vi "Test_MergeErrorsPublication_ErrorCluster_ErrorMerged.vi"(8 "error in (no error)":errorcluster, 11 "TestCase in":refnum<class "TestPublicationPolicy.lvclass">) -> (0 "error out":errorcluster, 3 "TestCase out":refnum<class "TestPublicationPolicy.lvclass">)   [LabVIEW 2017, in "TestPublicationPolicy.lvclass"]
uses:
  TestPublicationPolicy.lvclass
  MergeErrorsPublication/MergeErrorsPublication.lvclass
  C:/Git/mva-framework/Framework/IMediator/IPublicationPolicy/IPublicationPolicy.lvclass
  IMediator/IPublicationPolicy/IPublicationPolicy.lvclass
  Transport/QueueTransport/QueueTransport.lvclass/QueueTransport.ctl
  IMediator/PublishRequest/PublishRequest.lvclass/PublishRequest.ctl
  IMediator/MutexedPublishRequest/MutexedPublishRequest.lvclass/MutexedPublishRequest.ctl
  IMediator/PublishRequest/Write Publish Request Data.vi
  Transport/QueueTransport/QueueTransport.lvclass
  C:/Git/mva-framework/Framework/IMediator/ITransport/ITransport.lvclass
  IMediator/MutexedPublishRequest/MutexedPublishRequest.lvclass
  C:/Git/mva-framework/Framework/IMediator/PublishRequest/PublishRequest.lvclass
  <vilib>/Utility/error.llb/Error Cluster From Error Code.vi
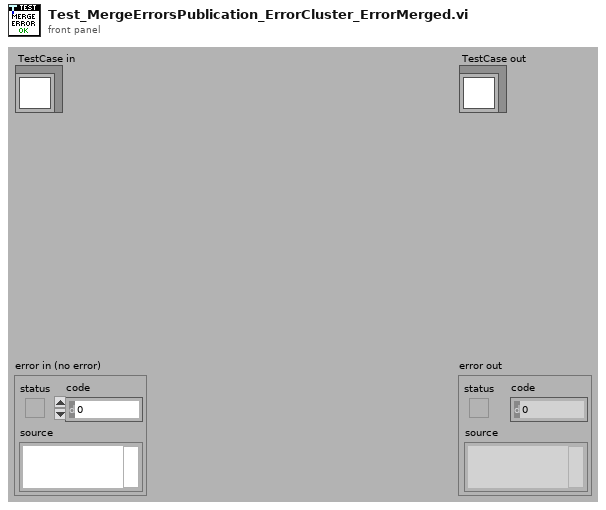
[diagram p1: front panel]
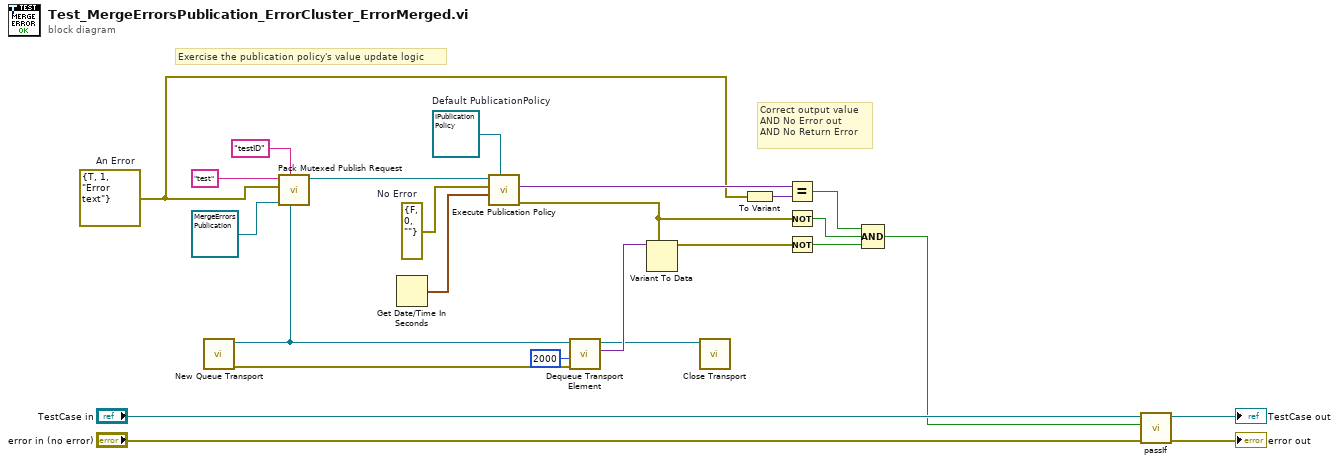
[diagram p0: block diagram]
diagram:
  w2 = errorcluster {"status"=TRUE, "code"=1, "source"="Error text"}  # An Error
  w17 = refnum<class "IPublicationPolicy.lvclass"> refnum  # Default PublicationPolicy
  w21 = errorcluster {"status"=FALSE, "code"=0, "source"=""}  # No Error
  # "Correct output value\nAND No Error out\nAND No Return Error"
  # "Exercise the publication policy's value update logic"
  n1 = call "New Queue Transport.vi"() -> ("error out"=w13:errorcluster, "QueueTransport"=w14:refnum<class "QueueTransport.lvclass">)  [unwired: 10 in]
  n2 = call "Pack Mutexed Publish Request.vi"("Return Error Transport"=w14, "Publisher ID"="testID", "PublicationPolicy"=refnum<class "MergeErrorsPublication.lvclass"> refnum ("PublicationPolicy.lvlib:MergeErrorsPublication.lvclass"), "Datum Value or Type"=w2, "Datum Name"="test") -> ("MutexedPublishRequest Out"=w19:refnum<class "MutexedPublishRequest.lvclass">)  [unwired: 6 in]
  n3 = Get Date/Time In Seconds() -> (seconds since 1Jan1904=w20:timestamp)
  n4 = call-dynamic "Execute Publication Policy.vi"("Default PublicationPolicy"=w17, "Last Publish Time"=w20, "Last Published Value"=w21, "MutexedPublishRequest"=w19) -> ("error out (Reject Publication)"=w4:errorcluster, "Value to Publish"=w10:variant)  [unwired: 5 in, 1 out]
  n5 = call "Dequeue Transport Element.vi"("error in (no error)"=w13, "Timeout In ms (-1)"=2000, "QueueTransport in"=w14) -> ("Data"=w11:variant, "QueueTransport out"=w7:refnum<class "QueueTransport.lvclass">)  [unwired: 5 in, 2 out]
  n6 = Variant To Data(type=w4, Variant=w11) -> (data=w8:errorcluster)  [unwired: 1 in, 1 out]
  n7 = call-dynamic "Close Transport.vi"("QueueTransport in"=w7) -> ()  [unwired: 10 in, 1 out]
  n8 = To Variant(anything=w2) -> (Variant=w9:variant)
  n9 = Equal?(x=w10, y=w9) -> (x = y?=w6:bool)
  n10 = Not(x=w4) -> (.not. x?=w3:bool)
  n11 = Not(x=w8) -> (.not. x?=w5:bool)
  n12 = Compound Arithmetic op=AND(w6, w3, w5) -> (w1:bool)
  n13 = call-dynamic "passIf.vi"("error in (no error)"="error in (no error)", "pass"=w1, "TestCase in"="TestCase in") -> ("error out"=→"error out":errorcluster, "TestCase out"=→"TestCase out":refnum<class "TestPublicationPolicy.lvclass">)  [unwired: 7 in]
